vi "Measurement UI.vi"() -> ()   [LabVIEW 2024, in "Broadband Generation UI.lvlib"]
uses:
  Broadband Generation UI.lvlib
  <vilib>/Utility/error.llb/Trim Whitespace One-Sided.vi
panel:
  in  "sample rate":dbl=51200.0 min=100.0 max=1000000.0 step=100.0 format="%#_g Hz"
  in  "output configurations":T1(array[cluster])=[{"channel"="Dev1/ao0", "range"=5.0, "terminal configuration"=-1, "broadband type"=0, "level"=0.5}] {"level" min=0.0 max=10.0 format="%_4g V"; "broadband type" items=["White Noise", "Pink Noise", "Periodic Random Noise", "Maximum Length Sequence"]; "terminal configuration" items=["Default"=-1, "RSE"=10083, "Differential"=10106, "Pseudodifferential"=12529]; "range" min=0.1 max=10.0 step=1.0 format="± %#_4g V"}
  in  "levels":dbl[](array[numeric])=[1.0, 1.0]
  in  "type":i32[](array[ring]) items=["White Noise", "Pink Noise", "Periodic Random Noise", "Maximum Length Sequence"]
  in  "terminal cfgs":i32[](array[numeric])=[-1, -1]
  in  "ranges":dbl[](array[numeric])=[3.16, 3.16]
  in  "physical channels":string[](array[string])=["Dev1/ao0", "Dev1/ao1"]
  out "error out":bool
  out "Task":u16(ring)
  out "generator status":string="Idle"
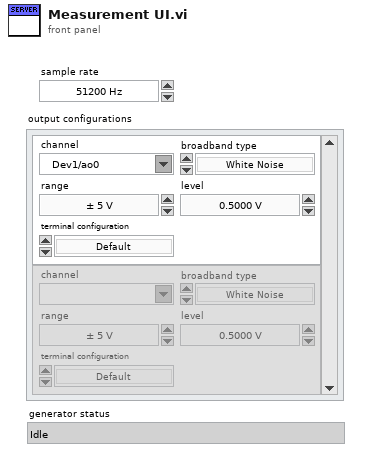
[diagram p1: front panel]
types:
  T1 = cluster{"channel":tag, "range":dbl, "terminal configuration":i32, "broadband type":i32, "level":dbl}[]
  T2 = cluster{"channel":tag, "range":dbl, "terminal configuration":i32, "broadband type":i32, "level":dbl}
  T3 = enum8{"Enabled", "Disabled", "Disabled and Grayed Out"}
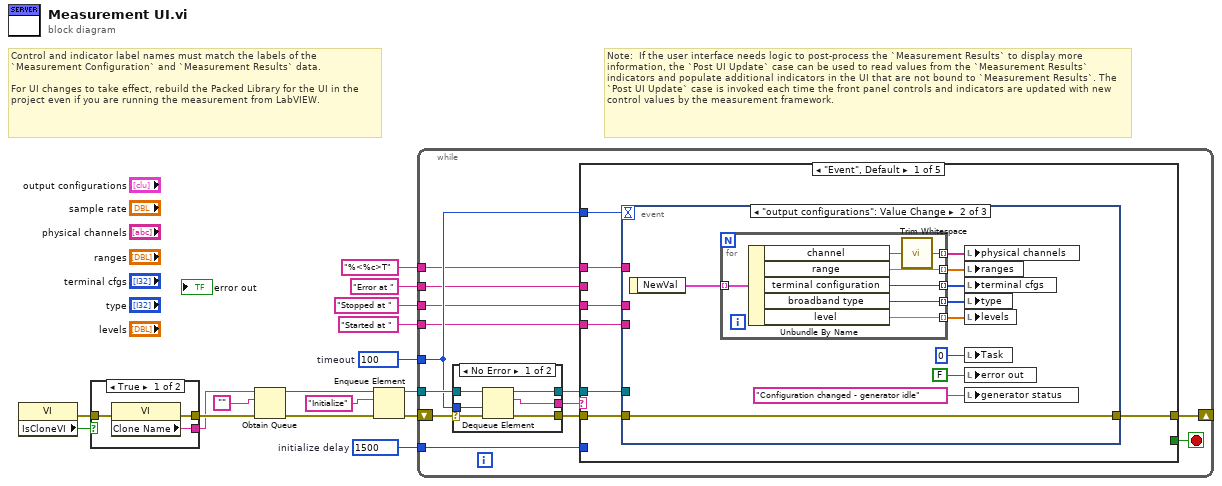
[diagram p0: block diagram]
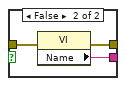
[diagram p2: hidden frame]
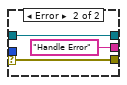
[diagram p3: hidden frame]
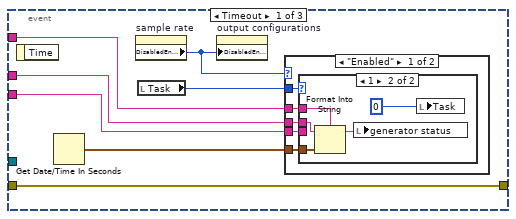
[diagram p4: hidden frame]
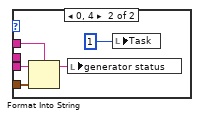
[diagram p7: hidden frame]
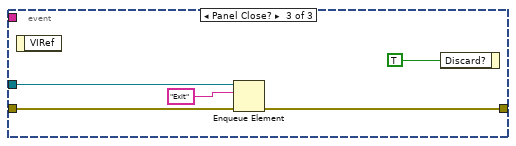
[diagram p8: hidden frame]
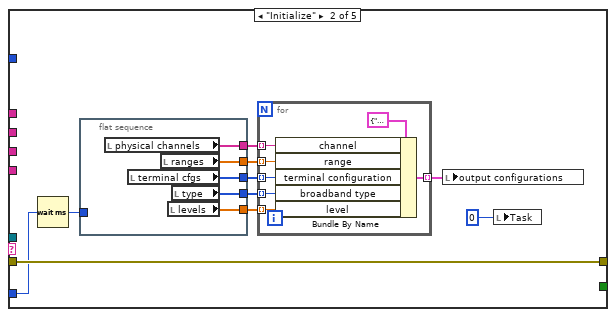
[diagram p9: hidden frame]
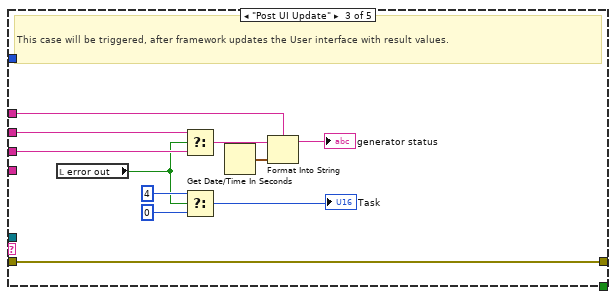
[diagram p10: hidden frame]
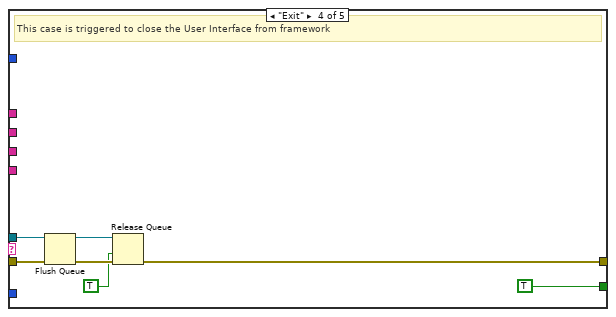
[diagram p11: hidden frame]
diagram:
  w1 = u32 1500  # initialize delay
  w6 = 100  # timeout
  # "Note:  If the user interface needs logic to post-process the `Measurement Results` to display more information, the `Post UI Update` case can be used to read values from the `Measurement Results` indicators and populate additional indicators in the UI that are not bound to `Measurement Results`. The `Post UI Update` case is invoked each time the front panel controls and indicators are updated with new control values by the measurement framework."
  # "Control and indicator label names must match the labels of the `Measurement Configuration` and `Measurement Results` data. \n\nFor UI changes to take effect, rebuild the Packed Library for the UI in the project even if you are running the measurement from LabVIEW."
  n1 = property class="VI"() -> (error out=w7:errorcluster, "IsCloneVI"=w8:bool)  [unwired: 2 in, 1 out]
  n2 = case shown="True" w8 {
    tunnel: [w19 w22] -> w16
    tunnel: [w18 w21] -> w15
    tunnel: w7 -> [w17 w20]
    frame True {
      n3 = property class="VI"(error in=w17) -> (error out=w19:errorcluster, "Clone Name"=w18:string)  [unwired: 1 in, 1 out]
    }
    frame False {
      n4 = property class="VI"(error in=w20) -> (error out=w22:errorcluster, "Name"=w21:string)  [unwired: 1 in, 1 out]
    }
  }
  n5 = Obtain Queue(name (unnamed)=w15, element data type="", error in (no error)=w16) -> (queue out=w12:refnum<queue>, error out=w14:errorcluster)  [unwired: 2 in, 1 out]
  n6 = Enqueue Element(queue=w12, element="Initialize", error in (no error)=w14) -> (queue out=w11:refnum<queue>, error out=w13:errorcluster)  [unwired: 1 in, 1 out]
  n7 = while {
    shift-right: [w30] -> _
    shift-left: w13 -> [w35]
    tunnel: w11 -> [w33]
    tunnel: w6 -> [w28]
    tunnel: "%<%c>T" ("format string") -> [w27]
    tunnel: "Error at " ("current status") -> [w26]
    tunnel: "Stopped at " ("current status") -> [w25]
    tunnel: "Started at " ("format string") -> [w24]
    tunnel: w1 -> [w23]
    stop <- w29 stop-if-true
    n8 = case shown="No Error" w35 {
      selector: w35 -> [w41 w44]
      tunnel: [w40 w44] -> w34
      tunnel: w33 -> [w39 w43]
      tunnel: [w38 w43] -> w32
      tunnel: [w37 "Handle Error"] -> w31
      tunnel: w28 -> [w36 _]
      frame No Error {
        n9 = Dequeue Element(queue=w39, timeout in ms (-1)=w36, error in (no error)=w41) -> (queue out=w38:refnum<queue>, element=w37:string, error out=w40:errorcluster)  [unwired: 1 out]
      }
      frame Error {
      }
    }
    n10 = case shown="\"Event\", Default" w31 {
      tunnel: w34 -> [w50 w110 w133 w140 w141]
      tunnel: w32 -> [w49 _ _ w138 _]
      tunnel: [w51 w110 w133 w135 w141] -> w30
      tunnel: [_ _ _ TRUE _] -> w29
      tunnel: w28 -> [w48 _ _ _ _]
      tunnel: w27 -> [w47 _ w128 _ _]
      tunnel: w26 -> [_ _ w127 _ _]
      tunnel: w25 -> [w45 _ w126 _ _]
      tunnel: w24 -> [w46 _ _ _ _]
      tunnel: w23 -> [_ w109 _ _ _]
      frame "Event", Default {
        n11 = event shown="[1] \"output configurations\": Value Change" {
          selector: _ -> [_ _ _]
          dyn-events: _ -> [_ _ _]
          timeout: w48 -> [_ _ _]
          tunnel: [w58 w79 w98] -> w51
          tunnel: w50 -> [w58 w79 w99]
          tunnel: w49 -> [_ _ w97]
          tunnel: w47 -> [w56 _ _]
          tunnel: w46 -> [w53 _ _]
          tunnel: w45 -> [w52 _ _]
          event Timeout {
            n12 = event-data() -> ()  [unwired: 1 in, 1 out]
            n13 = Get Date/Time In Seconds() -> (seconds since 1Jan1904=w54:timestamp)
            n14 = property on="sample rate" class="DigNum (strict)"() -> ("DisabledEnum"=w57:T3)  [unwired: 2 in, 2 out]
            n15 = local read "Task"() -> (w55:u16)
            n16 = property on="output configurations" class="Arr (strict)"("DisabledEnum"=w57) -> ()  [unwired: 2 in, 2 out]
            n17 = case shown="\"Enabled\"" w57 {
              tunnel: w55 -> [w63 w73]
              tunnel: w53 -> [w60 w72]
              tunnel: w56 -> [w62 w70]
              tunnel: w54 -> [w61 w71]
              tunnel: w52 -> [w59 w69]
              frame "Enabled" {
                n18 = case shown="1" w63 {
                  tunnel: w62 -> [_ w68]
                  tunnel: w61 -> [_ w67]
                  tunnel: w60 -> [_ _]
                  tunnel: w59 -> [_ w66]
                  frame Default {
                  }
                  frame 1 {
                    n19 = Format Into String(format string=w68, initial string=w66, w67) -> (resulting string=w64:string)  [unwired: 1 in, 1 out]
                    n20 = local write "generator status"(w64) -> ()
                    n21 = local write "Task"(u16 0 ("Task")) -> ()
                  }
                }
              }
              frame Default {
                n22 = case shown="Default" w73 {
                  tunnel: w72 -> [_ w78]
                  tunnel: w71 -> [_ w77]
                  tunnel: w70 -> [_ w76]
                  tunnel: w69 -> [_ _]
                  frame Default {
                  }
                  frame 0, 4 {
                    n23 = Format Into String(format string=w76, initial string=w78, w77) -> (resulting string=w74:string)  [unwired: 1 in, 1 out]
                    n24 = local write "generator status"(w74) -> ()
                    n25 = local write "Task"(u16 1 ("Task")) -> ()
                  }
                }
              }
            }
          }
          event "output configurations": Value Change {
            n26 = event-data() -> ("NewVal"=w88:T1)  [unwired: 1 in]
            n27 = for {
              tunnel: w88 -> [w95] mode=indexing
              tunnel: [w89] -> w87 mode=indexing
              tunnel: [w94] -> w86 mode=indexing
              tunnel: [w93] -> w85 mode=indexing
              tunnel: [w92] -> w84 mode=indexing
              tunnel: [w91] -> w83 mode=indexing
              n28 = Unbundle By Name(w95) -> ("channel"=w90:tag, "range"=w94:dbl, "terminal configuration"=w93:i32, "broadband type"=w92:i32, "level"=w91:dbl)
              n29 = call <vilib>:"Trim Whitespace.vi"("string"=w90) -> ("trimmed string"=w89:string)  [unwired: 1 in]
            }
            n30 = local write "physical channels"(w87) -> ()
            n31 = local write "ranges"(w86) -> ()
            n32 = local write "terminal cfgs"(w85) -> ()
            n33 = local write "type"(w84) -> ()
            n34 = local write "levels"(w83) -> ()
            n35 = local write "Task"(u16 0 ("Task")) -> ()
            n36 = local write "error out"(FALSE ("error out")) -> ()
            n37 = local write "generator status"("Configuration changed - generator idle" ("current status")) -> ()
          }
          event Panel Close? {
            n38 = event-data() -> ()  [unwired: 1 in, 1 out]
            n39 = Enqueue Element(queue=w97, element="Exit", error in (no error)=w99) -> (error out=w98:errorcluster)  [unwired: 1 in, 2 out]
            n40 = event-data("Discard?"=TRUE) -> ()  [unwired: 1 in, 1 out]
          }
        }
      }
      frame "Initialize" {
        n41 = Wait (ms)(milliseconds to wait=w109) -> (millisecond timer value=w102:u32)
        n42 = flat-sequence {
          tunnel: [w122] -> w108
          tunnel: [w121] -> w107
          tunnel: [w120] -> w106
          tunnel: [w119] -> w105
          tunnel: [w118] -> w104
          tunnel: w102 -> [_]
          frame #0 {
            n43 = local read "physical channels"() -> (w122:string[])
            n44 = local read "terminal cfgs"() -> (w120:i32[])
            n45 = local read "ranges"() -> (w121:dbl[])
            n46 = local read "levels"() -> (w118:dbl[])
            n47 = local read "type"() -> (w119:i32[])
          }
        }
        n48 = for {
          tunnel: w108 -> [w116] mode=indexing
          tunnel: w107 -> [w115] mode=indexing
          tunnel: w106 -> [w114] mode=indexing
          tunnel: w105 -> [w113] mode=indexing
          tunnel: w104 -> [w112] mode=indexing
          tunnel: [w111] -> w103 mode=indexing
          n49 = Bundle By Name(cluster=T2 {"channel"="Dev1/ao0", "range"=3.16, "terminal configuration"=-1, "broadband type"=0, "level"=1.0} ("output configuration"), "channel"=w116, "range"=w115, "terminal configuration"=w114, "broadband type"=w113, "level"=w112) -> (w111:T2)
        }
        n50 = local write "output configurations"(w103) -> ()
        n51 = local write "Task"(u16 0 ("Task")) -> ()
      }
      frame "Post UI Update" {
        # "This case will be triggered, after framework updates the User interface with result values."
        n52 = local read "error out"() -> (w125:bool)
        n53 = Select(t=w127, s=w125, f=w126) -> (s? t:f=w132:string)
        n54 = Select(t=u16 4 ("Task"), s=w125, f=u16 0 ("Task")) -> (s? t:f=→"Task":u16)
        n55 = Get Date/Time In Seconds() -> (seconds since 1Jan1904=w131:timestamp)
        n56 = Format Into String(format string=w128, initial string=w132, w131) -> (resulting string=→"generator status":string)  [unwired: 1 in, 1 out]
      }
      frame "Exit" {
        # "This case is triggered to close the User Interface from framework"
        n57 = Flush Queue(queue=w138, error in (no error)=w140) -> (queue out=w137:refnum<queue>, error out=w136:errorcluster)  [unwired: 1 out]
        n58 = Release Queue(queue=w137, force destroy? (F)=TRUE, error in (no error)=w136) -> (error out=w135:errorcluster)  [unwired: 2 out]
      }
      frame "Handle Error" {
      }
    }
  }
